vi "other_called_vis.vi"(8 "error in (no error)":errorcluster, 9 "options":T1={"Whole Hierarchy?"=TRUE, "Commented Out Diagrams?"=enum."Always include commented out diagrams", "Static VI Refs?"=TRUE, "Dynamic Dispatching?"=enum."No dynamic dispatch VIs", "Include Missing Items?"=FALSE, "Include Standard VIs?"=TRUE, "Include Reentrant Clones?"=enum."Include the clone VI", "Include Poly VIs?"=FALSE, "Include Global VIs?"=FALSE, "Include Control VIs?"=FALSE, "Include Generic VIs?"=FALSE, "Include Alternate Call Setups?"=FALSE, "Keep Express VIs?"=FALSE, "Load Block Diagram?"=FALSE}, 10 "name of caller in (you)":string) -> (0 "error out":errorcluster, 1 "vi paths":path[](array[path]), 2 "vi names":string[](array[string]))   [LabVIEW 2015]
doc: "Finds other VIs called by this VI's caller"
uses:
  <vilib>/regexp/Match Regular Expression.xnode
panel:
  # "This vi lists oter vi's called by the caller"
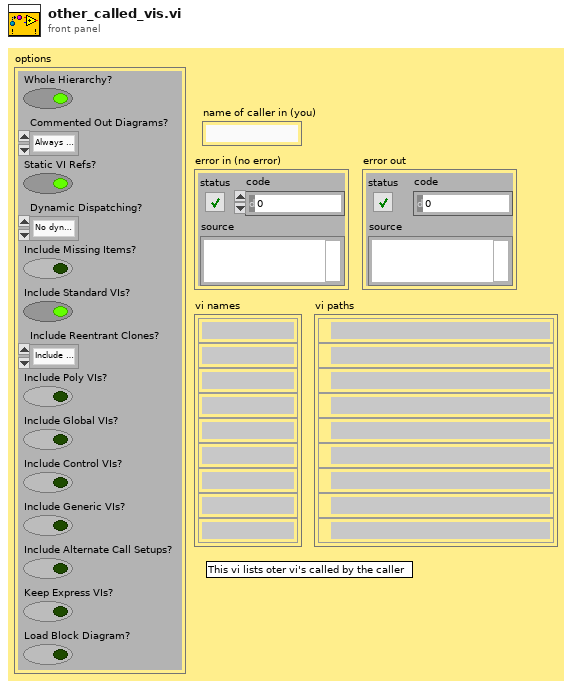
[diagram p1: front panel]
types:
  T1 = cluster{"Whole Hierarchy?":bool, "Commented Out Diagrams?":enum8{"Only include commented out diagrams if diagram already loaded", "Never include commented out diagrams", "Always include commented out diagrams"}, "Static VI Refs?":bool, "Dynamic Dispatching?":enum8{"No dynamic dispatch VIs", "Include nearest implementation", "Include all overrides"}, "Include Missing Items?":bool, "Include Standard VIs?":bool, "Include Reentrant Clones?":enum8{"Include the clone VI", "Include the original reentrant VI instead of the clone VI", "Include both the original reentrant VI and the clone VI"}, "Include Poly VIs?":bool, "Include Global VIs?":bool, "Include Control VIs?":bool, "Include Generic VIs?":bool, "Include Alternate Call Setups?":bool, "Keep Express VIs?":bool, "Load Block Diagram?":bool}
  T2 = enum8{"Only include commented out diagrams if diagram already loaded", "Never include commented out diagrams", "Always include commented out diagrams"}
  T3 = enum8{"No dynamic dispatch VIs", "Include nearest implementation", "Include all overrides"}
  T4 = enum8{"Include the clone VI", "Include the original reentrant VI instead of the clone VI", "Include both the original reentrant VI and the clone VI"}
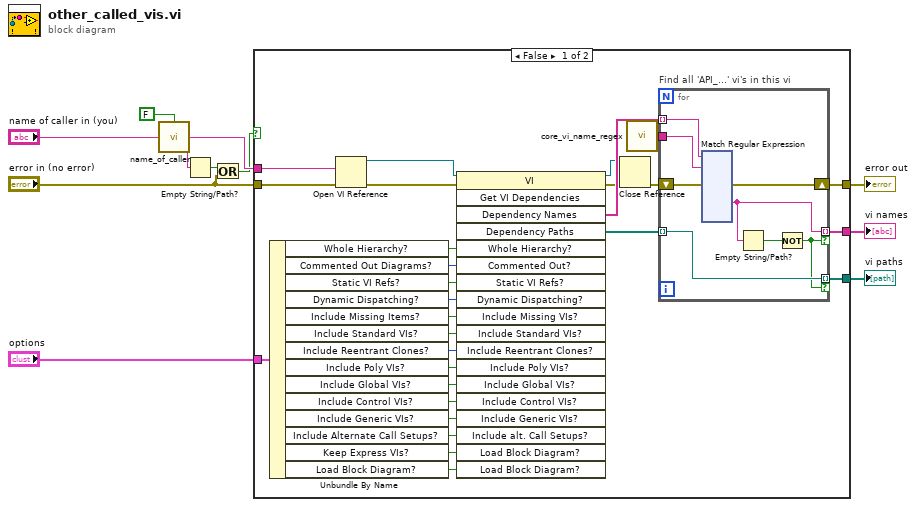
[diagram p0: block diagram]
diagram:
  n1 = call "name_of_caller.vi"("is in inlined vi? (F)"=FALSE, "name of caller in"="name of caller in (you)") -> ("name of caller out"=w6:string)  [unwired: 2 in]
  n2 = Empty String/Path?(string/path=w6) -> (empty?=w5:bool)
  n3 = Or(x=w5, y="error in (no error)") -> (x .or. y?=w3:bool)
  n4 = case shown="False" w3 {
    tunnel: "options" -> [w35 _]
    tunnel: [w15 w166] -> w7
    tunnel: w6 -> [w14 _]
    tunnel: "error in (no error)" -> [w13 w166]
    tunnel: [w12 _] -> w2
    tunnel: [w11 _] -> w1
    frame False {
      n5 = Unbundle By Name(w35) -> ("Whole Hierarchy?"=w34:bool, "Commented Out Diagrams?"=w33:T2, "Static VI Refs?"=w32:bool, "Dynamic Dispatching?"=w31:T3, "Include Missing Items?"=w30:bool, "Include Standard VIs?"=w29:bool, "Include Reentrant Clones?"=w28:T4, "Include Poly VIs?"=w27:bool, "Include Global VIs?"=w26:bool, "Include Control VIs?"=w25:bool, "Include Generic VIs?"=w24:bool, "Include Alternate Call Setups?"=w23:bool, "Keep Express VIs?"=w22:bool, "Load Block Diagram?"=w21:bool)
      n6 = Open VI Reference(vi path=w14, error in (no error)=w13) -> (vi reference=w20:refnum<vi>, error out=w19:errorcluster)  [unwired: 4 in]
      n7 = invoke class="VI" method="Get VI Dependencies"(reference=w20, error in=w19, "Whole Hierarchy?"=w34, "Commented Out?"=w33, "Static VI Refs?"=w32, "Dynamic Dispatching?"=w31, "Include Missing VIs?"=w30, "Include Standard VIs?"=w29, "Include Reentrant Clones?"=w28, "Include Poly VIs?"=w27, "Include Global VIs?"=w26, "Include Control VIs?"=w25, "Include Generic VIs?"=w24, "Include alt. Call Setups?"=w23, "Load Block Diagram?"=w22, "Load Block Diagram?"=w21) -> (reference out=w18:refnum<vi>, error out=w17:errorcluster, "Dependency Names"=w36:string[], "Dependency Paths"=w37:path[])  [unwired: 3 in, 15 out]
      n8 = Close Reference(reference=w18, error in (no error)=w17) -> (error out=w16:errorcluster)
      n9 = call "core_vi_name_regex.vi"() -> ("regex"=w38:string)
      n10 = for "Find all 'API_...' vi's in this vi" {
        tunnel: w38 -> [w46]
        tunnel: [w44] -> w11 mode=indexing if=w40
        tunnel: w37 -> [w44] mode=indexing
        tunnel: w36 -> [w45] mode=indexing
        shift-right: [w42] -> w15
        shift-left: w16 -> [w43]
        tunnel: [w39] -> w12 mode=indexing if=w40
        n11 = xnode "Match Regular Expression"("input string"=w45, "regular expression"=w46, "error in"=w43) -> ("error out"=w42:errorcluster, "submatch 2"=w39:string)  [unwired: 3 in, 7 out]
        n12 = Empty String/Path?(string/path=w39) -> (empty?=w41:bool)
        n13 = Not(x=w41) -> (.not. x?=w40:bool)
      }
    }
    frame True {
      # "Skip when no caller, or on error"
    }
  }
  "error out" <- w7
  "vi names" <- w2
  "vi paths" <- w1
